vi "Shooter_Winch1_18.vi"(4 "IsNotThereIn":bool, 6 "Winch Pot Location":dbl, 8 "LastIndex":dbl, 9 "three":bool, 10 "two":bool, 11 "one":bool) -> (0 "LastIndexOut":dbl, 1 "Winch Pot LocationOut":dbl, 3 "IsNotThere":bool)   [LabVIEW 2013]
panel:
  out "Winch Desired Location":dbl
  in  "Array":dbl[](array[numeric])
  out "Winch Motor Power Out":dbl
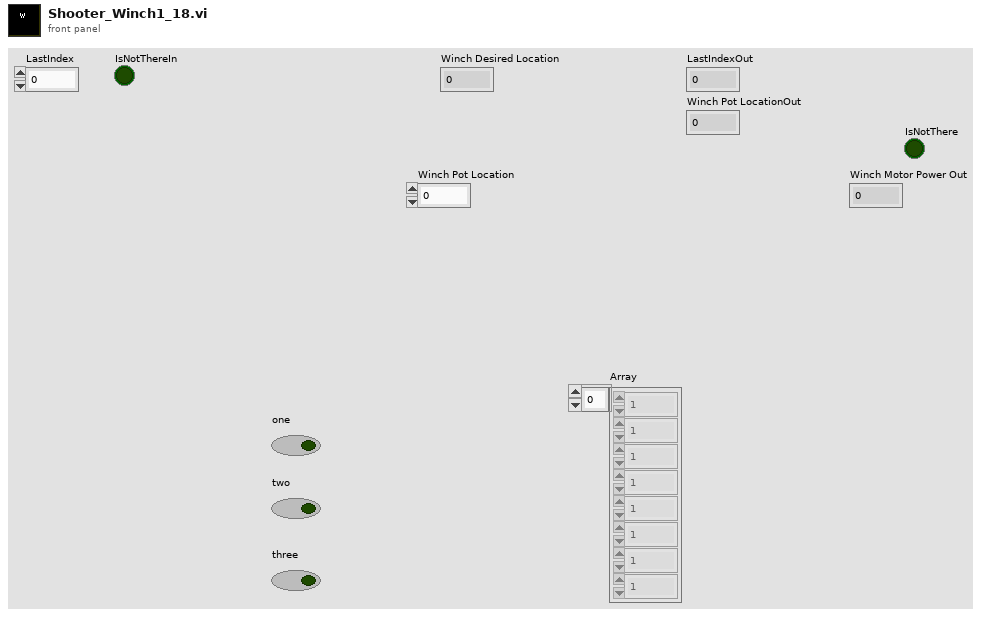
[diagram p1: front panel]
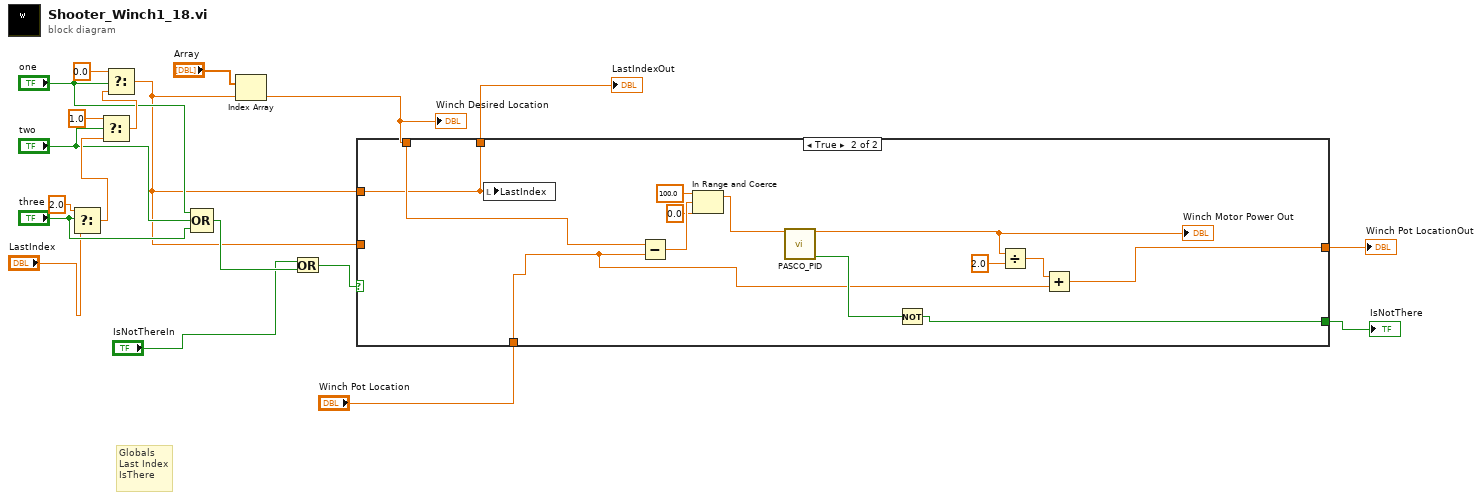
[diagram p0: block diagram]
diagram:
  # "Globals\nLast Index\nIsThere"
  n1 = Select(t=2.0, s="three", f="LastIndex") -> (s? t:f=w17:dbl)
  n2 = Select(t=1.0, s="two", f=w17) -> (s? t:f=w16:dbl)
  n3 = Select(t=0.0, s="one", f=w16) -> (s? t:f=w5:dbl)
  n4 = Compound Arithmetic op=OR("one", "two", "three") -> (w9:bool)
  n5 = Index Array(array="Array", index=w5) -> (element=w3:dbl)
  "Winch Desired Location" <- w3
  n6 = Or(x="IsNotThereIn", y=w9) -> (x .or. y?=w19:bool)
  n7 = case shown="True" w19 {
    tunnel: [_ w29] -> w18
    tunnel: w3 -> [_ w28]
    tunnel: w5 -> [_ _]
    tunnel: "Winch Pot Location" -> [w20 w27]
    tunnel: w5 -> [_ w25]
    tunnel: [w20 w26] -> w4
    tunnel: [_ w25] -> w1
    frame False {
    }
    frame True {
      n8 = local write "LastIndex"(w25) -> ()
      n9 = Subtract(x=w28, y=w27) -> (x-y=w24:dbl)
      n10 = In Range and Coerce(upper limit=100.0, x=w24, lower limit=0.0) -> (coerced(x)=w23:dbl)  [unwired: 1 out]
      n11 = call "PASCO_PID.vi"("Delta"=w23) -> ("Power Out"=w33:dbl, "IsThere"=w30:bool)  [unwired: 13 in]
      "Winch Motor Power Out" <- w33
      n12 = Not(x=w30) -> (.not. x?=w29:bool)
      n13 = Divide(x=w33, y=2.0) -> (x/y=w32:dbl)
      n14 = Add(x=w32, y=w27) -> (x+y=w26:dbl)
    }
  }
  "IsNotThere" <- w18
  "LastIndexOut" <- w1
  "Winch Pot LocationOut" <- w4
